vi "GLdrv_DATA_SAMP.vi"(0 "Connection ID":T2, 5 "Sampling":T1(ring), 11 "error in (no error)":errorcluster, 13 "Query(f)":bool) -> (4 "Connection ID Out":T2, 6 "Sampling out":T1(ring), 15 "error out":errorcluster)   [LabVIEW 2017, in "GL860_Driver.lvlib"]
doc: "サンプリング間隔の設定\n10/20/50/100/125/200/250/500(MS)/\n1/2/5/10/20/30/60/120/300/600/1200/1800/3600(S)\n例) :DATA:SAMP 500MS"
uses:
  GL860_Driver.lvlib
  ConnectionID.ctl
  GLdrv_RW.ctl
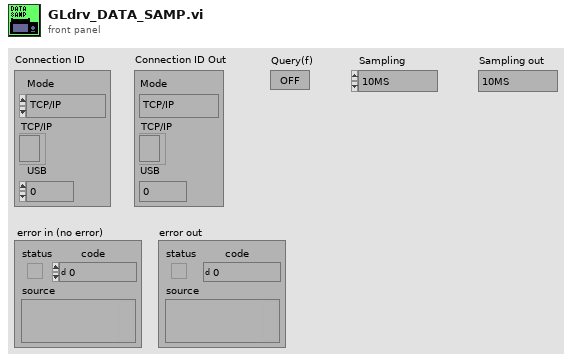
[diagram p1: front panel]
types:
  T1 = enum16{"10MS", "20MS", "50MS", "100MS", "125MS", "200MS", "250MS", "500MS", "1S", "2S", "5S", "10S", "20S", "30S", "60S", "120S", "300S", "600S", "1200S", "1800S", "3600S"}
  T2 = typedef "ConnectionID.ctl" = cluster{"Mode":enum16{"TCP/IP", "USB"}, "TCP/IP":refnum<k5>, "USB":i32}
  T3 = typedef "GLdrv_RW.ctl" = enum16{"Auto", "Read", "Write", "Buffer"}
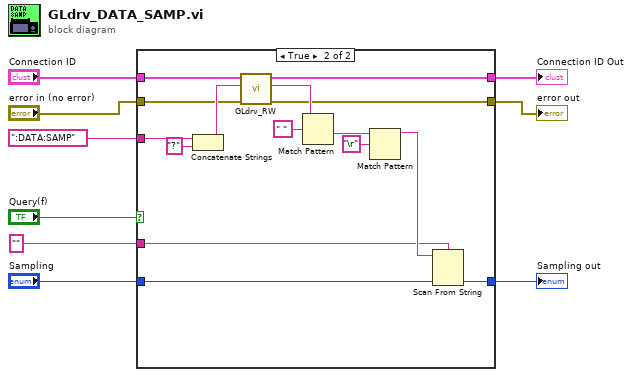
[diagram p0: block diagram]
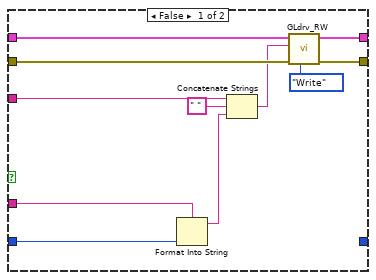
[diagram p2: hidden frame]
diagram:
  n1 = case shown="TRUE" "Query(f)" {
    tunnel: ":DATA:SAMP" ("Command") -> [w20 w32]
    tunnel: [w15 w24] -> w9
    tunnel: [w17 w28] -> w8
    tunnel: "Connection ID" -> [w18 w29]
    tunnel: "error in (no error)" -> [w16 w25]
    tunnel: "Sampling" -> [w11 w23]
    tunnel: [_ w22] -> w1
    tunnel: "" ("Param") -> [w10 w21]
    frame False {
      n2 = Format Into String(format string=w10, w11) -> (resulting string=w12:string)  [unwired: 2 in, 1 out]
      n3 = Concatenate Strings(w20, " " ("string"), w12) -> (w14:string)
      n4 = call "GLdrv_RW.vi"("Mode(read)"=GLdrv_RW."Write", "error in (no error)"=w16, "data in"=w14, "Connection ID"=w18) -> ("error out"=w15:errorcluster, "Connection ID Out"=w17:T2)  [unwired: 3 in, 3 out]
    }
    frame True {
      n5 = Concatenate Strings(w32, "?" ("string")) -> (w27:string)
      n6 = call "GLdrv_RW.vi"("error in (no error)"=w25, "data in"=w27, "Connection ID"=w29) -> ("error out"=w24:errorcluster, "data out"=w26:string, "Connection ID Out"=w28:T2)  [unwired: 4 in, 2 out]
      n7 = Match Pattern(string=w26, regular expression=" " ("search string/char (-)")) -> (after substring=w33:string)  [unwired: 4 out]
      n8 = Match Pattern(string=w33, regular expression="\r") -> (before substring=w30:string)  [unwired: 4 out]
      n9 = Scan From String(format string=w21, input string=w30, default 1=w23) -> (output 1=w22:T1)  [unwired: 2 in, 3 out]
    }
  }
  "Connection ID Out" <- w8
  "error out" <- w9
  "Sampling out" <- w1
